vi "AskandReply.vi"(10 "Send":string, 11 "VISA Refnum in":refnum<visa-resource-name>) -> (3 "Reply":string)   [LabVIEW 2020]
panel:
  in  "error in (no error)":errorcluster
  out "error out":errorcluster
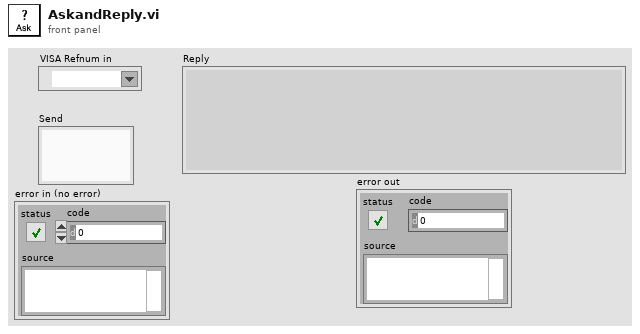
[diagram p1: front panel]
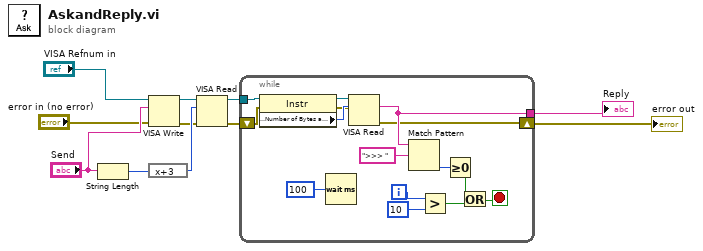
[diagram p0: block diagram]
diagram:
  n1 = String Length(string="Send") -> (length=w9:i32)
  n2 = VISA Write(VISA resource name="VISA Refnum in", write buffer="Send", error in (no error)="error in (no error)") -> (VISA resource name out=w6:refnum<visa-resource-name>, error out=w5:errorcluster)  [unwired: 1 out]
  n3 = expression code="x+3"(w9) -> (w10:i32)
  n4 = VISA Read(VISA resource name=w6, byte count=w10, error in (no error)=w5) -> (VISA resource name out=w11:refnum<visa-resource-name>, error out=w4:errorcluster)  [unwired: 2 out]
  n5 = while {
    tunnel: w11 -> [w26]
    tunnel: [w22] -> w1
    shift-right: [w12] -> w3
    shift-left: w4 -> [w14]
    i -> [w19]
    stop <- w15 stop-if-true
    n6 = property class="Instr"(reference=w26, error in=w14) -> (reference out=w24:refnum<visa-resource-name>, error out=w13:errorcluster, "Serial Settings:Number of Bytes at Serial Port"=w25:u32)
    n7 = Wait (ms)(milliseconds to wait=u32 100) -> ()  [unwired: 1 out]
    n8 = VISA Read(VISA resource name=w24, byte count=w25, error in (no error)=w13) -> (read buffer=w22:string, error out=w12:errorcluster)  [unwired: 2 out]
    n9 = Match Pattern(string=w22, regular expression=">>> ") -> (offset past match=w20:i32)  [unwired: 1 in, 3 out]
    n10 = Greater?(x=w19, y=10) -> (0:w16:bool)
    n11 = Greater Or Equal To 0?(x=w20) -> (x >= 0?=w17:bool)
    n12 = Or(x=w17, y=w16) -> (x .or. y?=w15:bool)
  }
  "Reply" <- w1
  "error out" <- w3
